vi "UA_Data_To_Item.vi"(1 "data":string) -> (0 "item":T1={"name"="", "data type"=1, "access level"=1, "description"=""} {"data type" items=["Boolean"=1, "SByte"=2, "Byte"=3, "Int16"=4, "UInt16"=5, "Int32"=6, "UInt32"=7, "Int64"=8, "UInt64"=9, "Float"=10, "Double"=11, "String"=12, "DateTime"=13, "ByteString"=15, "Array of Boolean"=101, "Array of SByte"=102, "Array of Byte"=103, "Array of Int16"=104, "Array of UInt16"=105, "Array of Int32"=106, "Array of UInt32"=107, "Array of Int64"=108, "Array of UInt64"=109, "Array of Float"=110, "Array of Double"=111, "Array of String"=112, "Array of DateTime"=113, "Array of ByteString"=115]; "access level" items=["read-only"=1, "write-only"=2, "read/write"=3]})   [LabVIEW 2013]
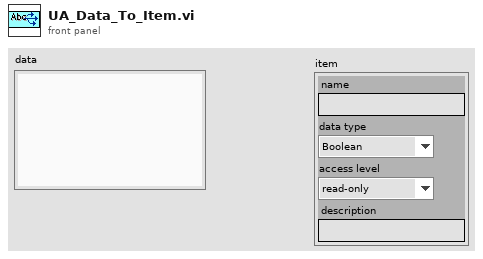
[diagram p1: front panel]
types:
  T1 = cluster{"name":string, "data type":u16, "access level":u16, "description":string}
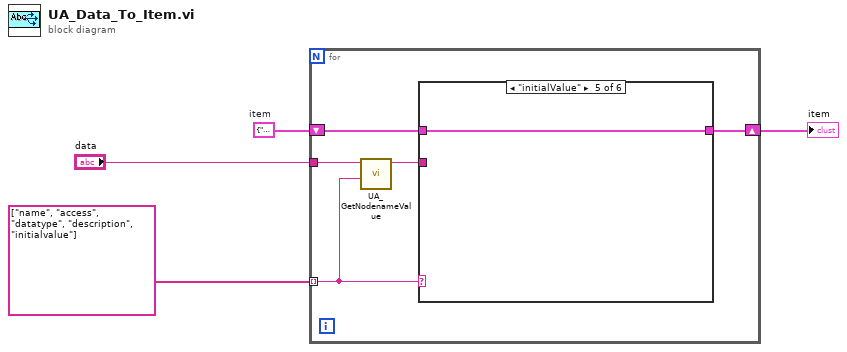
[diagram p0: block diagram]
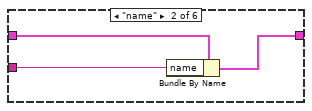
[diagram p3: hidden frame]
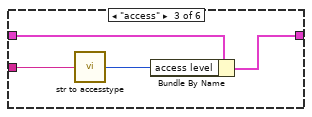
[diagram p4: hidden frame]
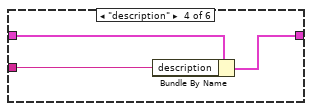
[diagram p5: hidden frame]
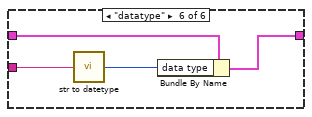
[diagram p6: hidden frame]
diagram:
  w1 = T1 {"name"="", "data type"=1, "access level"=1, "description"=""}  # item
  n1 = for {
    tunnel: "data" -> [w9]
    tunnel: string[] ["name", "access", "datatype", "description", "initialvalue"] -> [w8] mode=indexing
    shift-right: [w5] -> w2
    shift-left: w1 -> [w6]
    n2 = call "UA_GetNodenameValue.vi"("node name"=w8, "Data"=w9) -> ("value"=w7:string)  [unwired: 9 in]
    n3 = case shown="\"initialValue\"" w8 {
      tunnel: w7 -> [_ w11 w15 w18 _ w23]
      tunnel: w6 -> [w10 w13 w17 w20 w21 w25]
      tunnel: [w10 w12 w16 w19 w21 w24] -> w5
      frame Default {
      }
      frame "name" {
        n4 = Bundle By Name(cluster=w13, "name"=w11) -> (w12:T1)
      }
      frame "access" {
        n5 = call "str to accesstype.vi"("String"=w15) -> ("access level"=w14:u16)  [unwired: 6 in]
        n6 = Bundle By Name(cluster=w17, "access level"=w14) -> (w16:T1)
      }
      frame "description" {
        n7 = Bundle By Name(cluster=w20, "description"=w18) -> (w19:T1)
      }
      frame "initialValue" {
      }
      frame "datatype" {
        n8 = call "str to datetype.vi"("String"=w23) -> ("data type"=w22:u16)  [unwired: 5 in, 1 out]
        n9 = Bundle By Name(cluster=w25, "data type"=w22) -> (w24:T1)
      }
    }
  }
  "item" <- w2
